vi "U6 4-PWM.vi"(9 "Timer0/1 Duty Cycle [%]":dbl=50.0 format="%.1f", 10 "16-bit PWM Frequency [Hz]":dbl=40.0 format="%.2f") -> (2 "Actual 16-bit Frequency":dbl format="%.1f")   [LabVIEW 2021]
panel:
  in  "Timer/Counter Pin Offset":u8
  out "Update":bool
  out "Timer Value Array":u16[](array[numeric])
  in  "Timer2/3 Duty Cycle [%]":dbl=50.0 format="%.1f"
  in  "stop":bool
  out "Actual 8-bit Frequency":dbl format="%.1f"
  in  "FirstFound":bool=TRUE
  in  "Address":string="1"
  out "TimerClockDivisor":u8
  out "Error Message":string
  # "Demonstrates 2 channels of 16-bit PWM output and 2 channels of 8-bit PWM output.\nUses the 48 MHz divisor capable clock, and chooses a timer clock divisor to get\nas close as possible to the desired 16-bit PWM frequency.  Since a divisor capable\nclock is used, Counter0 is not available.  Since all timers use the same clock, the\nfrequency of the 8-bit PWM is fixed at 256 times the frequency of the 16-bit PWM.\nIf pin offset is 0, we get:\n\nFIO0 = PWM16, FIO1 = PWM16, FIO2 = PWM8, FIO3 = PWM8"
  # "Range is 2.86 to 732.42 Hz"
  # "This example allows the duty cycles to\nbe changed while the VI is running."
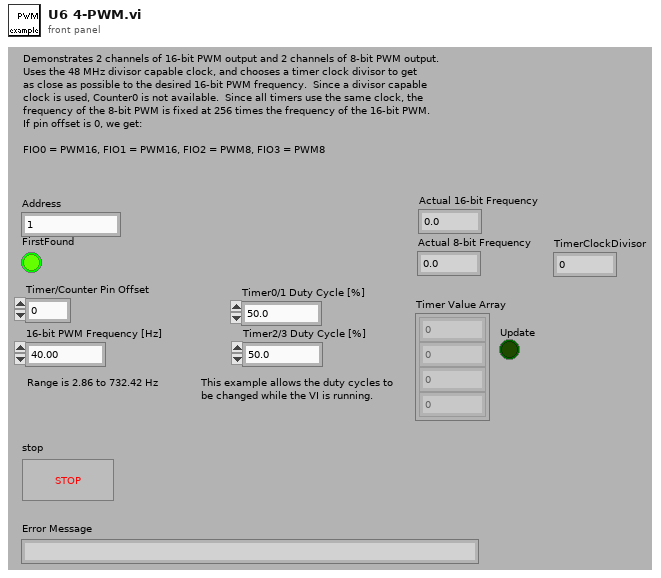
[diagram p1: front panel]
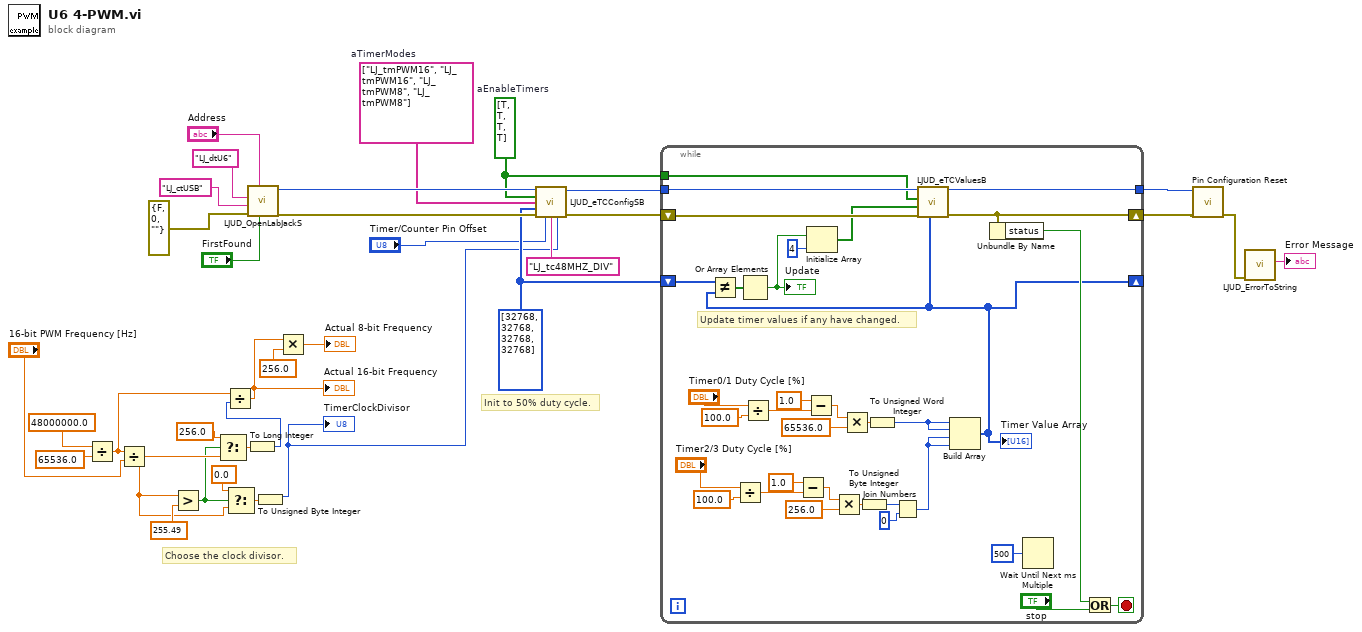
[diagram p0: block diagram]
diagram:
  w2 = bool[] [TRUE, TRUE, TRUE, TRUE]  # aEnableTimers
  w7 = string[] ["LJ_tmPWM16", "LJ_tmPWM16", "LJ_tmPWM8", "LJ_tmPWM8"]  # aTimerModes
  w6 = u16[] [32768, 32768, 32768, 32768] ("TimerValues")
  # "Choose the clock divisor."
  # "Init to 50% duty cycle."
  n1 = Divide(x=48000000.0, y=65536.0) -> (x/y=w22:dbl)
  n2 = Divide(x=w22, y="16-bit PWM Frequency [Hz]") -> (x/y=w26:dbl)
  n3 = Greater?(x=w26, y=255.49) -> (0:w25:bool)
  n4 = Select(t=256.0, s=w25, f=w26) -> (s? t:f=w28:dbl)
  n5 = Select(t=0.0, s=w25, f=w26) -> (s? t:f=w31:dbl)
  n6 = To Long Integer(number=w28) -> (32bit integer=w24:i32)
  n7 = Divide(x=w22, y=w24) -> (x/y=w21:dbl)
  "Actual 16-bit Frequency" <- w21
  n8 = call "LJUD_OpenLabJackS.vi"("FirstFound"="FirstFound", "Address"="Address", "error in"=errorcluster {"status"=FALSE, "code"=0, "source"=""}, "ConnectionType"="LJ_ctUSB", "DeviceType"="LJ_dtU6") -> ("error out"=w8:errorcluster, "Handle"=w9:i32)  [unwired: 4 in, 1 out]
  n9 = To Unsigned Byte Integer(number=w31) -> (unsigned 8bit integer=w3:u8)
  "TimerClockDivisor" <- w3
  n10 = Multiply(x=w21, y=256.0) -> (x*y=→"Actual 8-bit Frequency":dbl)
  n11 = call "LJUD_eTCConfigSB.vi"("Handle In"=w9, "aEnableTimers"=w2, "aTimerModes"=w7, "aTimerValues"=w6, "error in"=w8, "TCPinOffset"="Timer/Counter Pin Offset", "TimerClockBase"="LJ_tc48MHZ_DIV" ("Timer Clock Base"), "TimerClockDivisor"=w3) -> ("Handle Out"=w10:i32, "error out"=w11:errorcluster)  [unwired: 6 in]
  n12 = while {
    tunnel: w2 -> [w39]
    tunnel: [w44] -> w18
    shift-left: w6 -> [w51]
    shift-right: [w37] -> _
    tunnel: w10 -> [w41]
    shift-left: w11 -> [w42]
    shift-right: [w43] -> w17
    stop <- w52 stop-if-true
    # "Update timer values if any have changed."
    n13 = Divide(x="Timer2/3 Duty Cycle [%]", y=100.0) -> (x/y=w65:dbl)
    n14 = Divide(x="Timer0/1 Duty Cycle [%]", y=100.0) -> (x/y=w57:dbl)
    n15 = Subtract(x=1.0, y=w65) -> (x-y=w63:dbl)
    n16 = Subtract(x=1.0, y=w57) -> (x-y=w55:dbl)
    n17 = Multiply(x=w63, y=256.0) -> (x*y=w60:dbl)
    n18 = Multiply(x=w55, y=65536.0) -> (x*y=w54:dbl)
    n19 = To Unsigned Byte Integer(number=w60) -> (unsigned 8bit integer=w62:u8)
    n20 = To Unsigned Word Integer(number=w54) -> (unsigned 16bit integer=w35:u16)
    n21 = Join Numbers(hi=w62, lo=u8 0) -> ((hi.lo)=w36:u16)
    n22 = Build Array(w35, w35, w36, w36) -> (w37:u16[])
    "Timer Value Array" <- w37
    n23 = Not Equal?(x=w51, y=w37) -> (x != y?=w50:bool[])
    n24 = Or Array Elements(Boolean array=w50) -> (logical OR=w49:bool)
    "Update" <- w49
    n25 = Initialize Array(w49, 4 ("Dimension Size")) -> (w40:bool[])
    n26 = call "LJUD_eTCValuesB.vi"("aTimerValues Write"=w37, "error in"=w42, "aUpdateResetTimers"=w40, "aReadTimers"=w39, "Handle In"=w41) -> ("error out"=w43:errorcluster, "Handle Out"=w44:i32)  [unwired: 3 in, 2 out]
    n27 = Unbundle By Name(w43) -> ("status"=w48:bool)
    n28 = Wait Until Next ms Multiple(millisecond multiple=u32 500) -> ()  [unwired: 1 out]
    n29 = Or(x=w48, y="stop") -> (x .or. y?=w52:bool)
  }
  n30 = call "Pin Configuration Reset.vi"("error in"=w17, "Handle In"=w18) -> ("error out"=w16:errorcluster)  [unwired: 8 in, 1 out]
  n31 = call "LJUD_ErrorToString.vi"("error in"=w16) -> ("String"=→"Error Message":string)  [unwired: 10 in]
